vi "D-O Settings Dialog.vi"(8 "error in (no error)":errorcluster, 10 "Message Queues":T10, 11 "D-O Module State Cluster In":T4={"D-O Module Config"={"GUID"="", "Drop Coords"={"Horizontal"=0, "Vertical"=0}, "Process Name"="", "User name"="", "Queue Name"="", "Settings"={"Valve Settings"={"D-O Settings"={"DAQmx Task Name"="", "Output Channel"=0, "Output Channel Names"=[]}, "VICI Electronic Actuator"={"VISA resource name"="", "Mode"=enum."Two Positions With Stops", "Simulated"=FALSE}}, "Valve Type"=enum."Default", "Time On (Sec)"=0.0, "Time Off (Sec)"=0.0, "Run?"=FALSE}, "Load Count"=0}, "State"=enum."Idle", "Start Time"=timestamp(0 s since 1904-01-01), "Current Time"=timestamp(0 s since 1904-01-01), "First Iteration"=FALSE, "Data"={"Valve State"={"D-O Settings"={"DAQmx Task Name"="", "Output Channel"=0, "Output Channel Names"=[]}, "VICI Electronic Actuator"={"VISA resource name"="", "Mode"=enum."Two Positions With Stops", "Simulated"=FALSE}}}, "Process Name"="", "Queue Name"="", "Program On?"=FALSE} {"Data"."Valve State"."D-O Settings"."Output Channel" items=["Choose a Channel"]; "D-O Module Config"."Settings"."Valve Settings"."D-O Settings"."Output Channel" items=["Choose a Channel"]}) -> (0 "error out":errorcluster, 1 "Cancelled?":bool=TRUE, 2 "UI Refresh Needed?":bool, 3 "D-O Module Config Out":T5={"GUID"="", "Drop Coords"={"Horizontal"=0, "Vertical"=0}, "Process Name"="", "User name"="", "Queue Name"="", "Settings"={"Valve Settings"={"D-O Settings"={"DAQmx Task Name"="", "Output Channel"=0, "Output Channel Names"=[]}, "VICI Electronic Actuator"={"VISA resource name"="", "Mode"=enum."Two Positions With Stops", "Simulated"=FALSE}}, "Valve Type"=enum."Digital Output Valve", "Time On (Sec)"=0.0, "Time Off (Sec)"=0.0, "Run?"=FALSE}, "Load Count"=0} {"Settings"."Valve Settings"."D-O Settings"."Output Channel" items=["Choose a Channel"]})   [LabVIEW 2018, in "D-O Module.lvlib"]
doc: "Dialog for selecting user specified settings."
uses:
  D-O Module.lvlib
  All Message Queues.ctl
  support/Message Queue/Message Cluster.ctl
  D-O Module Config Cluster.ctl
  <vilib>/Utility/miscctls.llb/LVPoint32TypeDef.ctl
  Valve Clusters.ctl
  D-O Module Settings Cluster.ctl
  D-O Device Settings Cluster.ctl
  VICI Electronic Actuator/VICI Electronic Actuator Settings.ctl
  D-O Module State Cluster.ctl
  Measure Instrument/State Enum.ctl
  support/Message Queue/Enqueue Message (Single).vi
  <vilib>/Utility/xml.llb/Write to XML File(string).vi
  Settings/Settings.lvlib
  <resource>/objmgr/daqmx.rc
  support/Message Queue/Message Queue.lvlib
  DIO Valve/VICI Electronic Actuator.lvlib
  Measure Instrument/Feed Module Engine.lvlib
panel:
  in  "Start":bool
  in  "Stop":bool
  in  "Settings Dialog":T3 {"D-O Settings"."Output Channel" items=["Choose a Channel"]}
  out "Channels":string[](array[string])
  in  "Cancel Button":bool
  in  "OK Button":bool
  # "Non visible portion of dialog (needed for connector pane)."
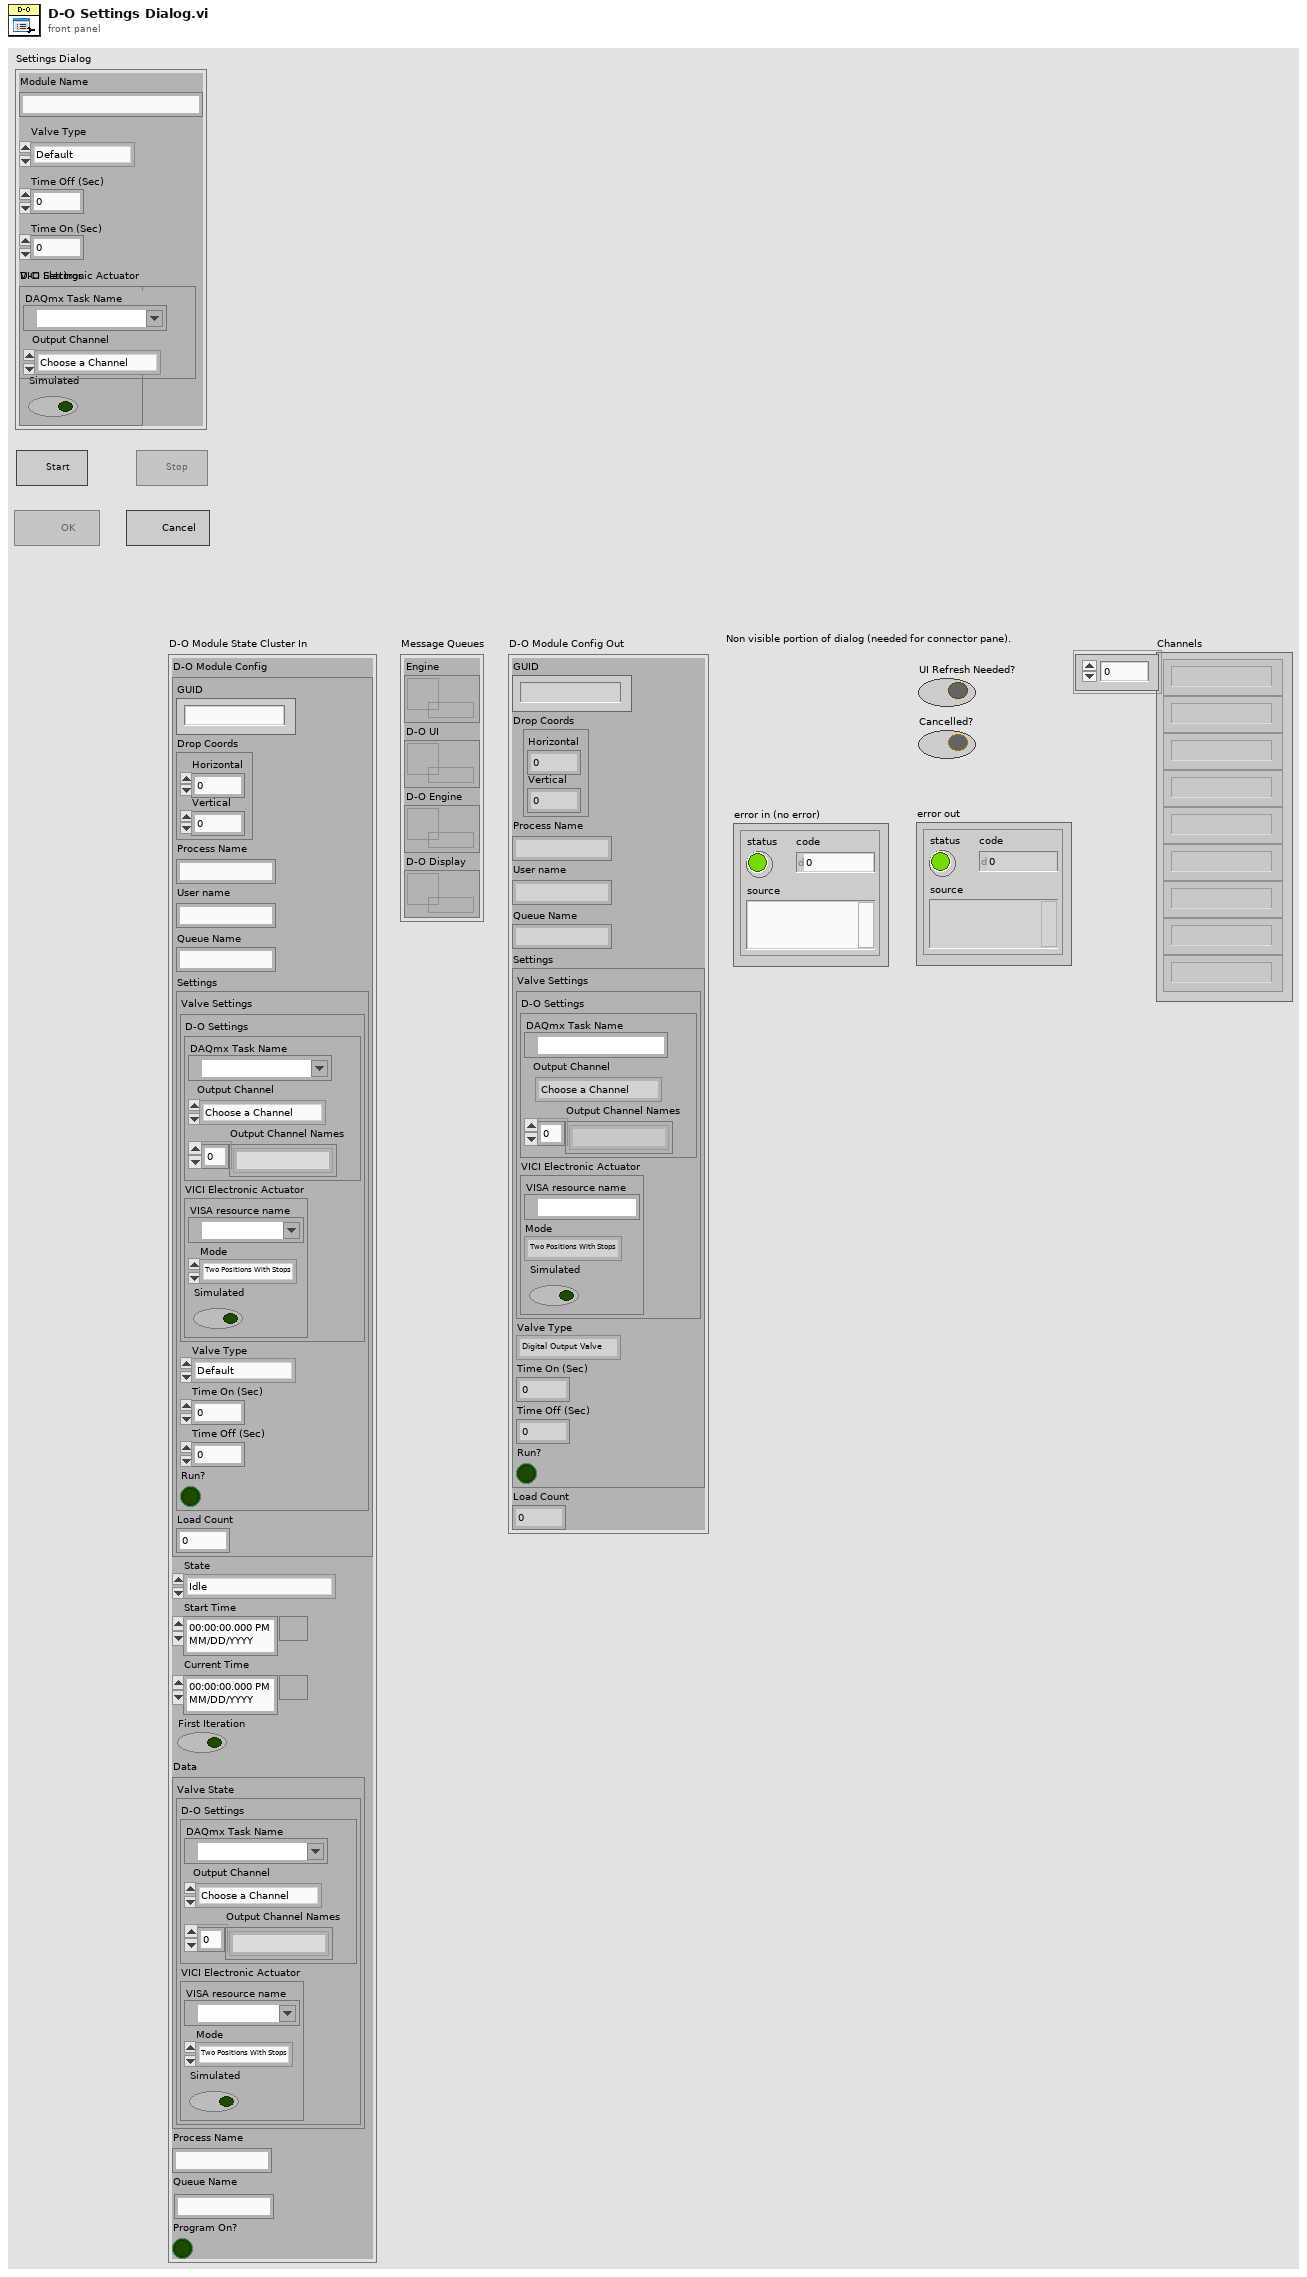
[diagram p1: front panel]
types:
  T1 = typedef "D-O Module.lvlib/D-O Device Settings Cluster.ctl" = cluster{"DAQmx Task Name":refnum<k21>, "Output Channel":u16, "Output Channel Names":string[]}
  T2 = typedef "VICI Electronic Actuator.lvlib/VICI Electronic Actuator Settings.ctl" = cluster{"VISA resource name":refnum<visa-resource-name>, "Mode":enum16{"Two Positions With Stops", "Two Positions Without Stops", "Mutiposition"}, "Simulated":bool}
  T3 = cluster{"Module Name":string, "Time Off (Sec)":dbl, "Time On (Sec)":dbl, "Valve Type":enum16{"Default", "Digital Output Valve", "VICI Electronic Actuator"}, "D-O Settings":T1, "VICI Electronic Actuator":T2}
  T4 = typedef "D-O Module.lvlib/D-O Module State Cluster.ctl" = cluster{"D-O Module Config":T5, "State":T9, "Start Time":timestamp, "Current Time":timestamp, "First Iteration":bool, "Data":cluster{"Valve State":T8}, "Process Name":string, "Queue Name":string, "Program On?":bool}
  T5 = typedef "D-O Module.lvlib/D-O Module Config Cluster.ctl" = cluster{"GUID":string, "Drop Coords":T6, "Process Name":string, "User name":string, "Queue Name":string, "Settings":T7, "Load Count":i32}
  T6 = typedef "LVPoint32TypeDef.ctl" = cluster{"Horizontal":i32, "Vertical":i32}
  T7 = typedef "D-O Module.lvlib/Valve Clusters.ctl" = cluster{"Valve Settings":T8, "Valve Type":enum16{"Default", "Digital Output Valve", "VICI Electronic Actuator"}, "Time On (Sec)":dbl, "Time Off (Sec)":dbl, "Run?":bool}
  T8 = typedef "D-O Module.lvlib/D-O Module Settings Cluster.ctl" = cluster{"D-O Settings":T1, "VICI Electronic Actuator":T2}
  T9 = typedef "Feed Module.lvlib/Feed Module Engine.lvlib/State Enum.ctl" = enum16{"Measuring", "Idle", "Paused"}
  T10 = typedef "D-O Module.lvlib/All Message Queues.ctl" = cluster{"Engine":refnum<queue>, "D-O UI":refnum<queue>, "D-O Engine":refnum<queue>, "D-O Display":refnum<queue>}
  T11 = enum16{"Default", "Digital Output Valve", "VICI Electronic Actuator"}
  T12 = enum8{"Enabled", "Disabled", "Disabled and Grayed Out"}
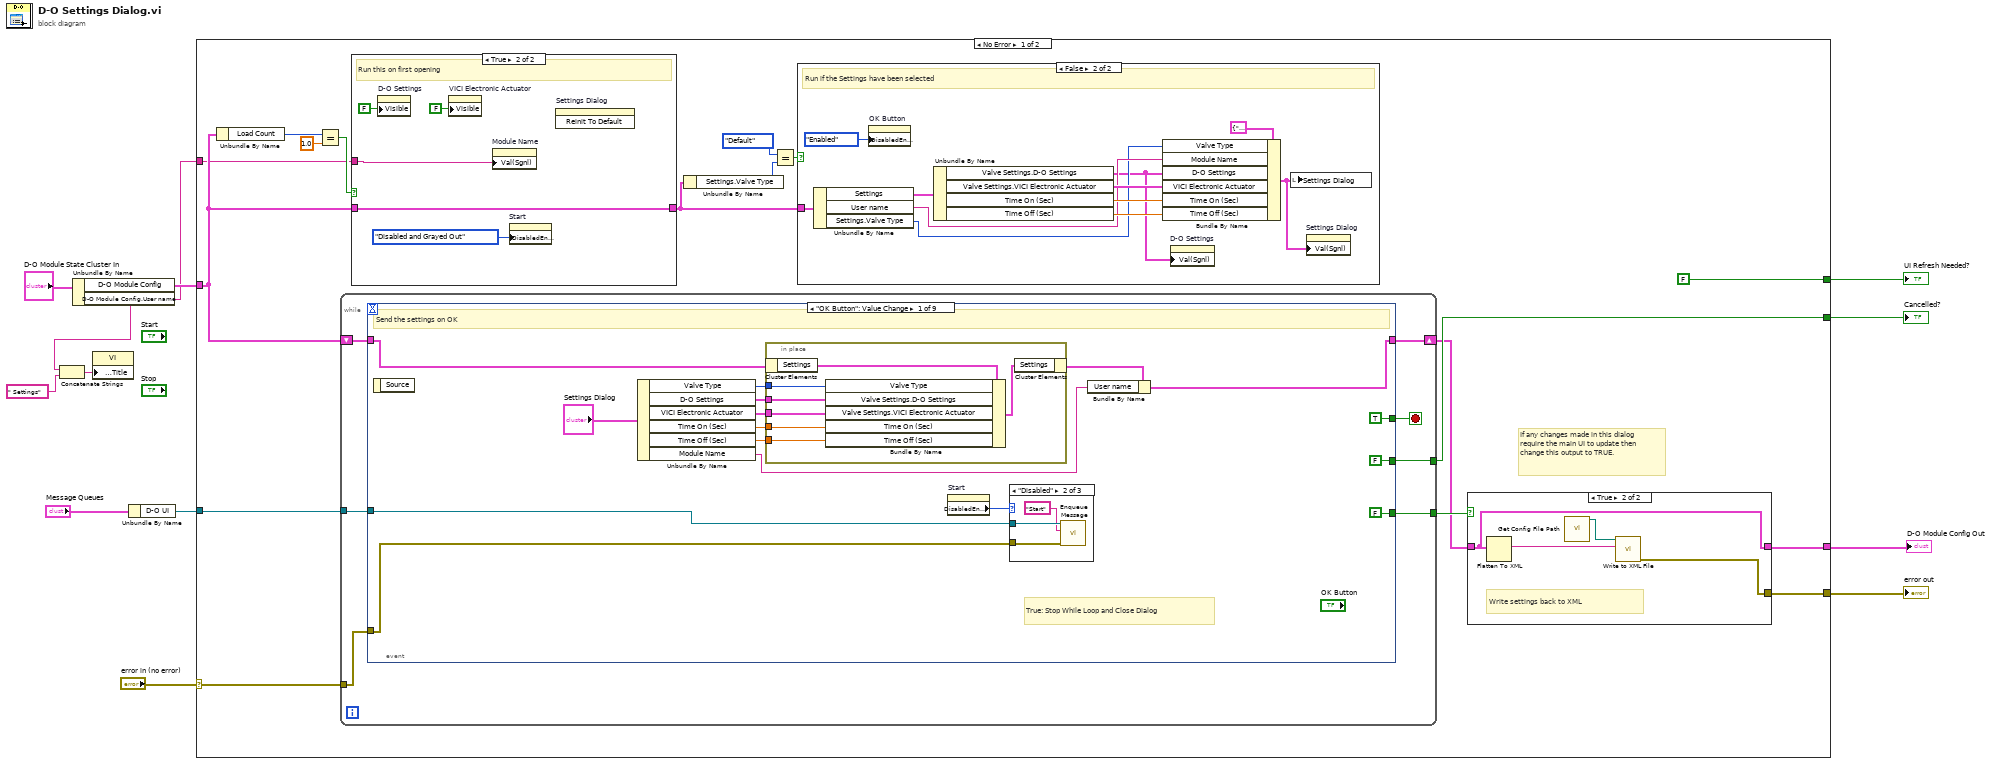
[diagram p0: block diagram]
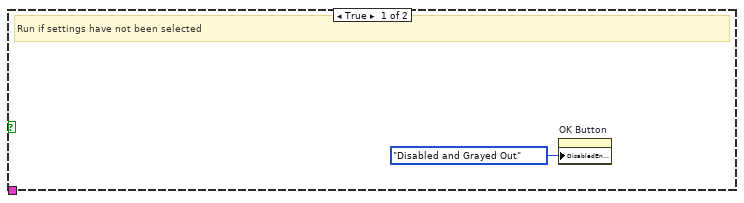
[diagram p2: hidden frame]
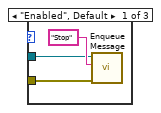
[diagram p4: hidden frame]
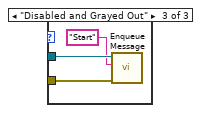
[diagram p5: hidden frame]
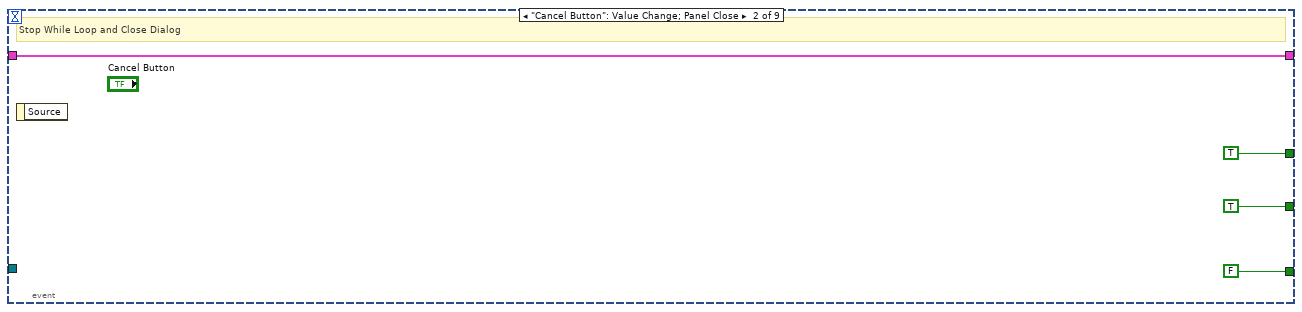
[diagram p6: hidden frame]
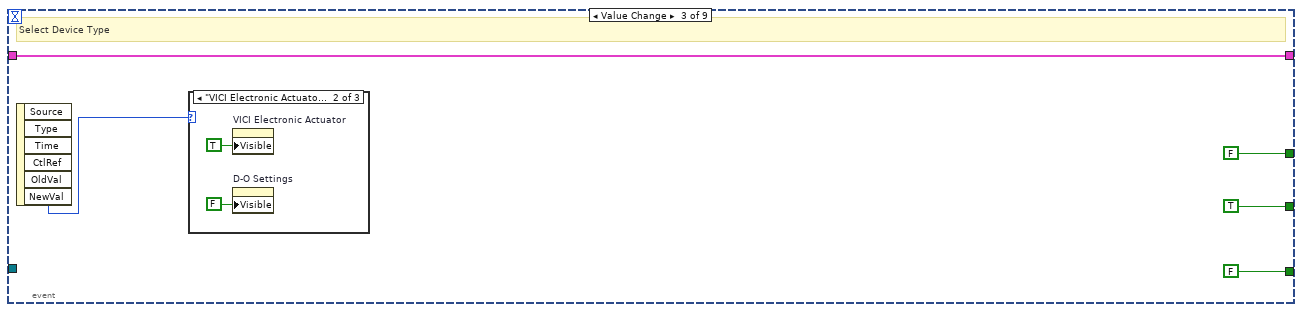
[diagram p7: hidden frame]
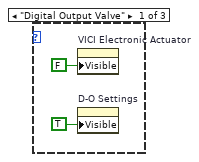
[diagram p8: hidden frame]
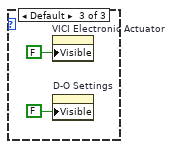
[diagram p9: hidden frame]
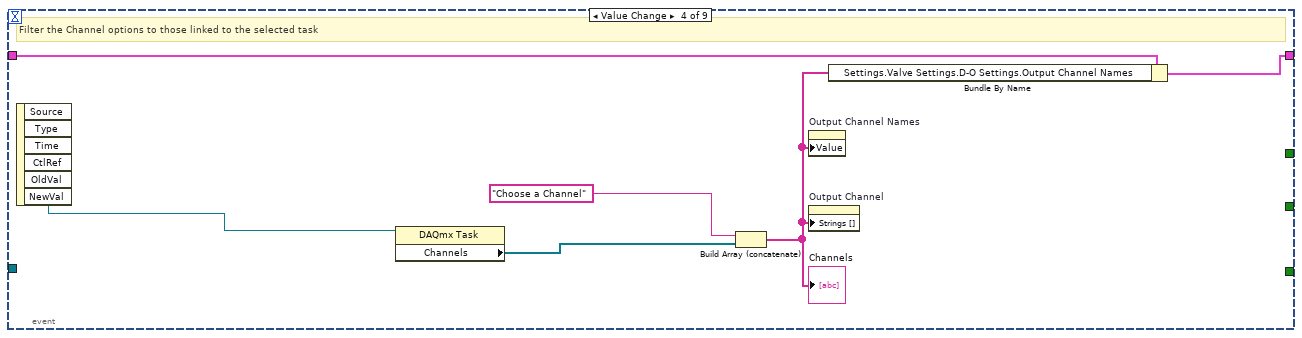
[diagram p10: hidden frame]
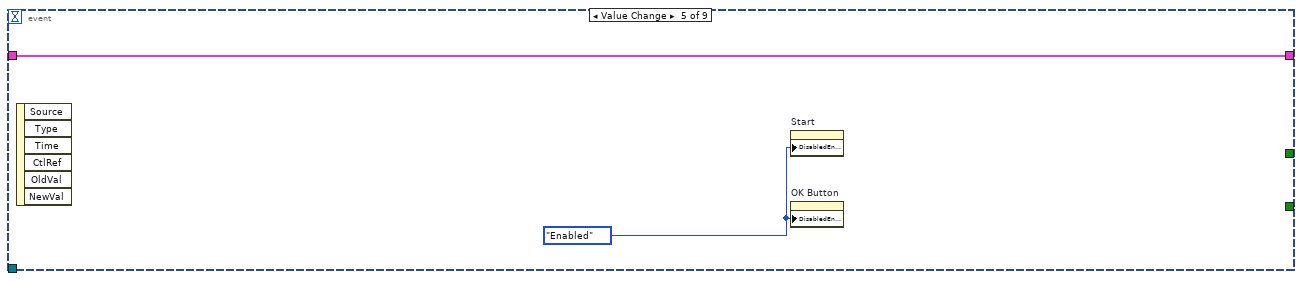
[diagram p11: hidden frame]
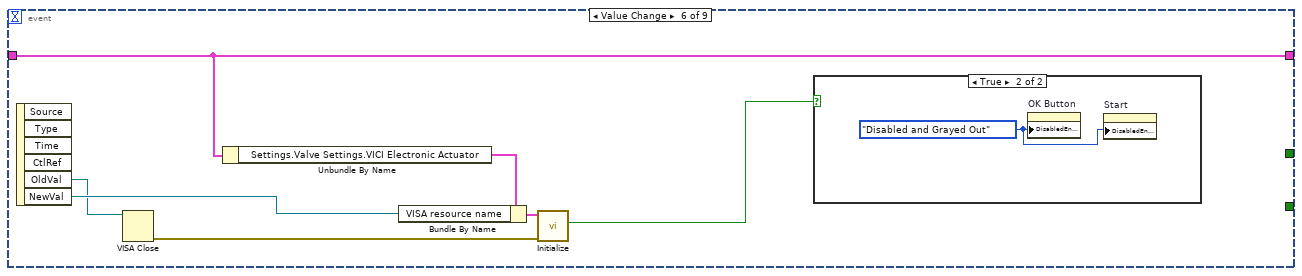
[diagram p12: hidden frame]
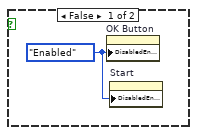
[diagram p13: hidden frame]
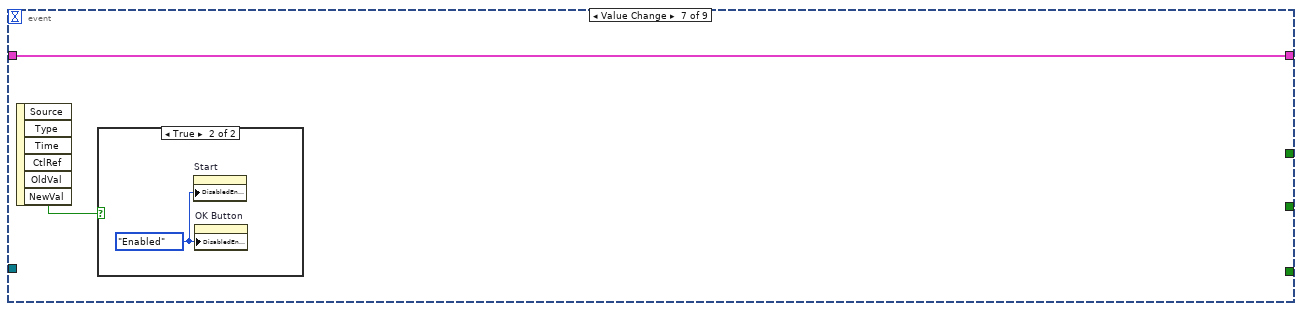
[diagram p14: hidden frame]
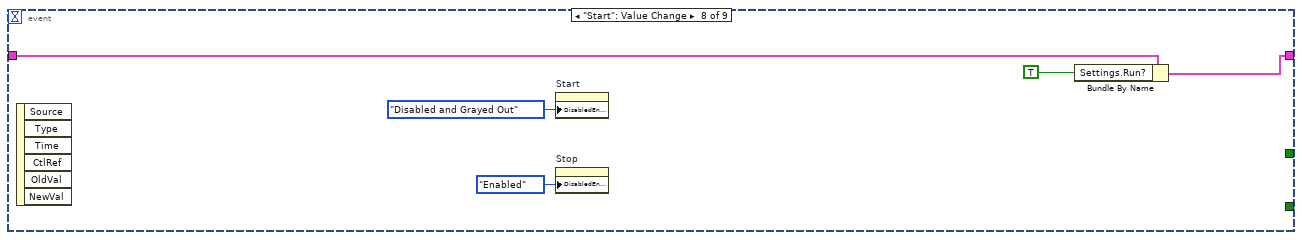
[diagram p16: hidden frame]
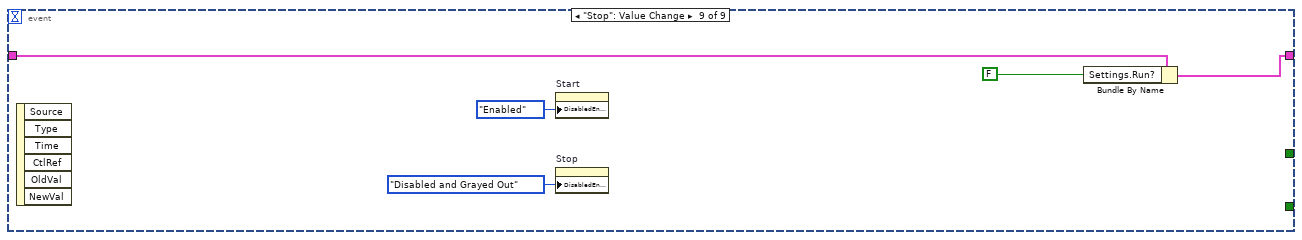
[diagram p17: hidden frame]
diagram:
  n1 = Unbundle By Name("D-O Module State Cluster In") -> ("D-O Module Config"=w4:T5, "D-O Module Config.User name"=w1:string)
  n2 = Concatenate Strings(w1, " Settings" ("string")) -> (w3:string)
  n3 = property class="VI"("Front Panel.Title"=w3) -> ()  [unwired: 2 in, 2 out]
  n4 = Unbundle By Name("Message Queues") -> ("D-O UI"=w9:refnum<queue>)
  n5 = case shown="No Error" "error in (no error)" {
    selector: "error in (no error)" -> [w24 w139]
    tunnel: [w26 w139] -> w12
    tunnel: w4 -> [w17 w137]
    tunnel: [w27 w137] -> w6
    tunnel: [FALSE ("UI Refresh Needed?") _] -> w11
    tunnel: [w28 TRUE ("UI Refresh Needed?")] -> w10
    tunnel: w9 -> [w25 _]
    tunnel: w1 -> [w13 _]
    frame No Error {
      # "If any changes made in this dialog require the main UI to update then change this output to TRUE."
      n6 = Unbundle By Name(w17) -> ("Load Count"=w23:i32)
      n7 = Equal?(x=w23, y=1.0) -> (x = y?=w20:bool)
      n8 = while {
        tunnel: [w54] -> w19
        tunnel: [w52] -> w28
        tunnel: w25 -> [w50]
        tunnel: w24 -> [w49]
        shift-right: [w51] -> w18
        shift-left: w17 -> [w48]
        stop <- w53 stop-if-true
        n9 = event shown="[0] \"OK Button\": Value Change" {
          selector: _ -> [_ _ _ _ _ _ _ _ _]
          dyn-events: _ -> [_ _ _ _ _ _ _ _ _]
          timeout: _ -> [_ _ _ _ _ _ _ _ _]
          tunnel: [FALSE ("UI Refresh Needed?") FALSE ("UI Refresh Needed?") FALSE ("UI Refresh Needed?") _ _ _ _ _ _] -> w54
          tunnel: [TRUE TRUE FALSE _ _ _ _ _ _] -> w53
          tunnel: [FALSE ("UI Refresh Needed?") TRUE ("UI Refresh Needed?") TRUE ("UI Refresh Needed?") _ _ _ _ _ _] -> w52
          tunnel: w48 -> [w61 w87 w92 w104 w109 w116 w120 w124 w128]
          tunnel: [w67 w87 w92 w103 w109 w116 w120 w123 w127] -> w51
          tunnel: w50 -> [w66 _ _ _ _ _ _ _ _]
          tunnel: w49 -> [w65 _ _ _ _ _ _ _ _]
          event "OK Button": Value Change {
            # "True: Stop While Loop and Close Dialog"
            # "Send the settings on OK"
            n10 = event-data() -> ()  [unwired: 1 in, 1 out]
            n11 = Unbundle By Name("Settings Dialog") -> ("Valve Type"=w60:T11, "D-O Settings"=w59:T1, "VICI Electronic Actuator"=w58:T2, "Time On (Sec)"=w57:dbl, "Time Off (Sec)"=w56:dbl, "Module Name"=w62:string)
            n12 = in-place {
              in-place-border: w60 -> [w76]
              in-place-border: w59 -> [w75]
              in-place-border: w58 -> [w74]
              in-place-border: w57 -> [w73]
              in-place-border: w56 -> [w72]
              n13 = in-place-cluster #1(w61) -> ("Settings"=w77:T7)
              n14 = Bundle By Name(cluster=w77, "Valve Type"=w76, "Valve Settings.D-O Settings"=w75, "Valve Settings.VICI Electronic Actuator"=w74, "Time On (Sec)"=w73, "Time Off (Sec)"=w72) -> (w71:T7)
              n15 = in-place-cluster #1("Settings"=w71) -> (w55:T5)
            }
            n16 = property on="Start" class="Bool"() -> ("DisabledEnum"=w64:T12)  [unwired: 2 in, 2 out]
            n17 = case shown="\"Disabled\"" w64 {
              tunnel: w66 -> [w79 w83 w86]
              tunnel: w65 -> [w78 w82 w85]
              frame "Enabled", Default {
                n18 = call-poly "Enqueue Message.vi"("error in (no error)"=w78, "Message"="Stop", "Message Queue"=w79) -> ()  [unwired: 7 in, 2 out]
              }
              frame "Disabled" {
                n19 = call-poly "Enqueue Message.vi"("error in (no error)"=w82, "Message"="Start", "Message Queue"=w83) -> ()  [unwired: 7 in, 2 out]
              }
              frame "Disabled and Grayed Out" {
                n20 = call-poly "Enqueue Message.vi"("error in (no error)"=w85, "Message"="Start", "Message Queue"=w86) -> ()  [unwired: 7 in, 2 out]
              }
            }
            n21 = Bundle By Name(cluster=w55, "User name"=w62) -> (w67:T5)
          }
          event "Cancel Button": Value Change; Panel Close {
            # "Stop While Loop and Close Dialog"
            n22 = event-data() -> ()  [unwired: 1 in, 1 out]
          }
          event "Settings Dialog.Valve Type": Value Change {
            # "Select Device Type"
            n23 = event-data() -> ("NewVal"=w91:T11)  [unwired: 1 in, 5 out]
            n24 = case shown="\"VICI Electronic Actuator\"" w91 {
              frame "Digital Output Valve" {
                n25 = property on="VICI Electronic Actuator" class="Clust (strict)"("Visible"=FALSE) -> ()  [unwired: 2 in, 2 out]
                n26 = property on="D-O Settings" class="Clust (strict)"("Visible"=TRUE) -> ()  [unwired: 2 in, 2 out]
              }
              frame "VICI Electronic Actuator" {
                n27 = property on="VICI Electronic Actuator" class="Clust (strict)"("Visible"=TRUE) -> ()  [unwired: 2 in, 2 out]
                n28 = property on="D-O Settings" class="Clust (strict)"("Visible"=FALSE) -> ()  [unwired: 2 in, 2 out]
              }
              frame Default {
                n29 = property on="VICI Electronic Actuator" class="Clust (strict)"("Visible"=FALSE) -> ()  [unwired: 2 in, 2 out]
                n30 = property on="D-O Settings" class="Clust (strict)"("Visible"=FALSE) -> ()  [unwired: 2 in, 2 out]
              }
            }
          }
          event Value Change {
            # "Filter the Channel options to those linked to the selected task"
            n31 = event-data() -> ("NewVal"=w107:refnum<k21>)  [unwired: 1 in, 5 out]
            n32 = property class="DAQmx Task"(reference=w107) -> ("Channels"=w105:refnum<k21>[])  [unwired: 1 in, 2 out]
            n33 = Build Array (concatenate)("Choose a Channel", w105) -> (w102:string[])
            "Channels" <- w102
            n34 = property on="Output Channel Names" class="Arr (strict)"("Value"=w102) -> ()  [unwired: 2 in, 2 out]
            n35 = property on="Output Channel" class="Ring (strict)"("Strings []"=w102) -> ()  [unwired: 2 in, 2 out]
            n36 = Bundle By Name(cluster=w104, "Settings.Valve Settings.D-O Settings.Output Channel Names"=w102) -> (w103:T5)
          }
          event Value Change {
            w108 = T12."Enabled" ("Disabled")
            n37 = event-data() -> ()  [unwired: 1 in, 6 out]
            n38 = property on="Start" class="Bool"("DisabledEnum"=w108) -> ()  [unwired: 2 in, 2 out]
            n39 = property on="OK Button" class="Bool"("DisabledEnum"=w108) -> ()  [unwired: 2 in, 2 out]
          }
          event Value Change {
            n40 = event-data() -> ("OldVal"=w111:refnum<visa-resource-name>, "NewVal"=w114:refnum<visa-resource-name>)  [unwired: 1 in, 4 out]
            n41 = VISA Close(VISA resource name=w111) -> (error out=w110:errorcluster)  [unwired: 1 in]
            n42 = Unbundle By Name(w116) -> ("Settings.Valve Settings.VICI Electronic Actuator"=w115:T2)
            n43 = Bundle By Name(cluster=w115, "VISA resource name"=w114) -> (w113:T2)
            n44 = call "Initialize.vi"("error in (no error)"=w110, "VICI Electronic Actuator In"=w113) -> ("No Valve Connected"=w112:bool)  [unwired: 6 in, 3 out]
            n45 = case shown="True" w112 {
              frame False {
                w117 = T12."Enabled" ("Disabled")
                n46 = property on="OK Button" class="Bool"("DisabledEnum"=w117) -> ()  [unwired: 2 in, 2 out]
                n47 = property on="Start" class="Bool"("DisabledEnum"=w117) -> ()  [unwired: 2 in, 2 out]
              }
              frame True {
                w118 = T12."Disabled and Grayed Out" ("Disabled")
                n48 = property on="OK Button" class="Bool"("DisabledEnum"=w118) -> ()  [unwired: 2 in, 2 out]
                n49 = property on="Start" class="Bool"("DisabledEnum"=w118) -> ()  [unwired: 2 in, 2 out]
              }
            }
          }
          event Value Change {
            n50 = event-data() -> ("NewVal"=w119:bool)  [unwired: 1 in, 5 out]
            n51 = case shown="True" w119 {
              frame False {
              }
              frame True {
                w121 = T12."Enabled" ("Disabled")
                n52 = property on="Start" class="Bool"("DisabledEnum"=w121) -> ()  [unwired: 2 in, 2 out]
                n53 = property on="OK Button" class="Bool"("DisabledEnum"=w121) -> ()  [unwired: 2 in, 2 out]
              }
            }
          }
          event "Start": Value Change {
            n54 = event-data() -> ()  [unwired: 1 in, 6 out]
            n55 = property on="Start" class="Bool"("DisabledEnum"=T12."Disabled and Grayed Out" ("Disabled")) -> ()  [unwired: 2 in, 2 out]
            n56 = property on="Stop" class="Bool"("DisabledEnum"=T12."Enabled" ("Disabled")) -> ()  [unwired: 2 in, 2 out]
            n57 = Bundle By Name(cluster=w124, "Settings.Run?"=TRUE) -> (w123:T5)
          }
          event "Stop": Value Change {
            n58 = event-data() -> ()  [unwired: 1 in, 6 out]
            n59 = property on="Start" class="Bool"("DisabledEnum"=T12."Enabled" ("Disabled")) -> ()  [unwired: 2 in, 2 out]
            n60 = property on="Stop" class="Bool"("DisabledEnum"=T12."Disabled and Grayed Out" ("Disabled")) -> ()  [unwired: 2 in, 2 out]
            n61 = Bundle By Name(cluster=w128, "Settings.Run?"=FALSE) -> (w127:T5)
          }
        }
      }
      n62 = case shown="True" w20 {
        tunnel: w17 -> [w42 w43]
        tunnel: [w42 w43] -> w21
        tunnel: w13 -> [_ w44]
        frame False {
        }
        frame True {
          # "Run this on first opening"
          n63 = property on="D-O Settings" class="Clust (strict)"("Visible"=FALSE) -> ()  [unwired: 2 in, 2 out]
          n64 = property on="VICI Electronic Actuator" class="Clust (strict)"("Visible"=FALSE) -> ()  [unwired: 2 in, 2 out]
          n65 = property on="Module Name" class="Str"("Val(Sgnl)"=w44) -> ()  [unwired: 2 in, 2 out]
          n66 = property on="Start" class="Bool"("DisabledEnum"=T12."Disabled and Grayed Out" ("Disabled")) -> ()  [unwired: 2 in, 2 out]
          n67 = invoke on="Settings Dialog" class="Clust (strict)" method="Reinit To Default"() -> ()  [unwired: 3 in, 3 out]
        }
      }
      n68 = Unbundle By Name(w21) -> ("Settings.Valve Type"=w16:T11)
      n69 = Equal?(x=T11."Default", y=w16) -> (x = y?=w14:bool)
      n70 = case shown="False" w14 {
        tunnel: w21 -> [_ w40]
        frame True {
          # "Run if settings have not been selected"
          n71 = property on="OK Button" class="Bool"("DisabledEnum"=T12."Disabled and Grayed Out" ("Disabled")) -> ()  [unwired: 2 in, 2 out]
        }
        frame False {
          # "Run if the Settings have been selected"
          n72 = Unbundle By Name(w40) -> ("Settings"=w41:T7, "User name"=w34:string, "Settings.Valve Type"=w33:T11)
          n73 = property on="OK Button" class="Bool"("DisabledEnum"=T12."Enabled" ("Disabled")) -> ()  [unwired: 2 in, 2 out]
          n74 = Unbundle By Name(w41) -> ("Valve Settings.D-O Settings"=w31:T1, "Valve Settings.VICI Electronic Actuator"=w39:T2, "Time On (Sec)"=w38:dbl, "Time Off (Sec)"=w37:dbl)
          n75 = Bundle By Name(cluster=T3 {"Module Name"="", "Time Off (Sec)"=0.0, "Time On (Sec)"=0.0, "Valve Type"=enum."Default", "D-O Settings"={"DAQmx Task Name"="", "Output Channel"=0, "Output Channel Names"=[]}, "VICI Electronic Actuator"={"VISA resource name"="", "Mode"=enum."Two Positions With Stops", "Simulated"=FALSE}} ("Settings Dialog"), "Valve Type"=w33, "Module Name"=w34, "D-O Settings"=w31, "VICI Electronic Actuator"=w39, "Time On (Sec)"=w38, "Time Off (Sec)"=w37) -> (w32:T3)
          n76 = property on="D-O Settings" class="Clust (strict)"("Val(Sgnl)"=w31) -> ()  [unwired: 2 in, 2 out]
          n77 = local write "Settings Dialog"(w32) -> ()
          n78 = property on="Settings Dialog" class="Clust (strict)"("Val(Sgnl)"=w32) -> ()  [unwired: 2 in, 2 out]
        }
      }
      n79 = case shown="True" w19 {
        tunnel: w18 -> [w132 w133]
        tunnel: [_ w134] -> w26
        tunnel: [w132 w133] -> w27
        frame False {
        }
        frame True {
          # "Write settings back to XML"
          n80 = Flatten To XML(anything=w133) -> (xml string=w135:string)
          n81 = call "Get Config File Path.vi"() -> ("XML File Path"=w136:path)  [unwired: 10 in, 1 out]
          n82 = call-poly <vilib>:"Write to XML File.vi"("XML Input"=w135, "XML File Path"=w136) -> ("error out"=w134:errorcluster)  [unwired: 7 in, 2 out]
        }
      }
    }
    frame Error {
    }
  }
  "UI Refresh Needed?" <- w11
  "error out" <- w12
  "Cancelled?" <- w10
  "D-O Module Config Out" <- w6
